vi "Uninit.vi"(11 "VMR Actor in":refnum<class "VMR Actor.lvclass">) -> (3 "VMR Actor out":refnum<class "VMR Actor.lvclass">)   [LabVIEW 2022 SP3, in "VMR Server.lvlib" / "VMR Actor.lvclass"]
doc: "This method is the inverse of the Pre Launch Init.vi. This method is called unconditionally at the end of an actor's lifetime, even if there was an error in Pre Launch Init.vi. Note that the self Enqueuer for the actor is already invalid by the time this VI executes: within this method, the actor may send messages to its caller but not to itself. This method executes before Last Ack is sent.\n\nThis method neither receives nor produces an error cluster. It is designed to provide an unconditional release of acquired resources. Any error raised during release is considered to be irrelevant to the actor's lifetime. If the actor truly needs to report some error status, it may send a message to caller or include information within itself that callers can examine when handling Last Ack."
uses:
  VMR Actor.lvclass
  <vilib>/ActorFramework/Actor/Actor.lvclass
  VMR Actor.lvclass/VMR Actor.ctl
  <vilib>/IlluminatedG/IG VoicemeeterRemote API/VoiceMeeterRemote/VoiceMeeterRemote/VoiceMeeterRemote.lvclass
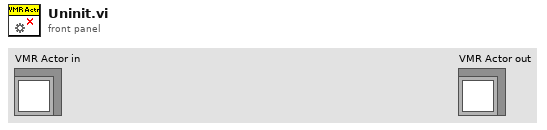
[diagram p1: front panel]
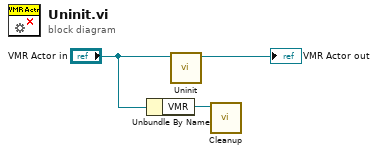
[diagram p0: block diagram]
diagram:
  n1 = Unbundle By Name("VMR Actor in") -> ("VMR"=w1:refnum<class "VoiceMeeterRemote.lvclass">)
  n2 = call-parent "Uninit.vi"("Actor in"="VMR Actor in") -> ("Actor out"=→"VMR Actor out":refnum<class "VMR Actor.lvclass">)  [unwired: 10 in]
  n3 = call <vilib>:"Cleanup.vi"("VoiceMeeterRemote in"=w1) -> ()  [unwired: 10 in, 1 out]
